vi "18.DMA-FIFO-2通道.vi"() -> ()   [LabVIEW 2019]
uses:
  <vilib>/rvi/Emulation/niFpgaGetClockAttributes.vi
  <vilib>/rvi/Emulation/niFpgaSctlEmulationGetInTimedLoop.vi
  <vilib>/rvi/Emulation/niFpgaEmulationReportErrorSimple.vi
  <vilib>/rvi/eio/common/nirviEmuTemplateMethod_errors.vi
  <vilib>/rvi/interface/RandomDataEmulation/niFpgaRandomDataHandleErrors.vi
  <vilib>/rvi/Emulation/niFpgaProcessEmulError.vi
  <vilib>/rvi/Emulation/niFpgaCriticalErrorInLSC.vi
  <vilib>/eio/EIONode/EIONode.xnode
  <vilib>/rvi/DataTransferAndStorage/Container/XNode/niFpgaContainer.xnode
  <vilib>/rvi/interface/RandomDataEmulation/nirviRandomDataFpgaReadWriteTemplate.vi
panel:
  in  "stop":bool
  in  "DMA Cleared?":bool
  out "Overflow?":bool
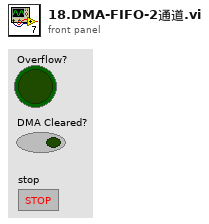
[diagram p1: front panel]
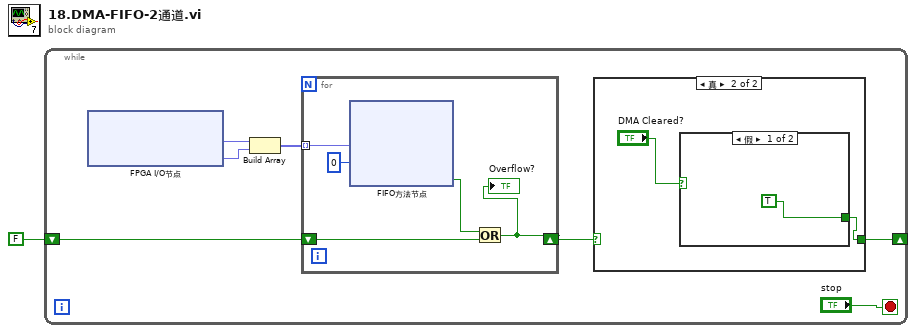
[diagram p0: block diagram]
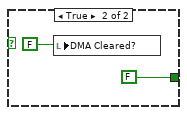
[diagram p3: hidden frame]
diagram:
  n1 = while {
    shift-right: [w3] -> _
    shift-left: FALSE -> [w5]
    stop <- "stop" stop-if-true
    n2 = xnode "FPGA I/O节点"() -> ("ConnectorB/AI0"=w8:fxp<+/-,24,5>, "ConnectorB/AI1"=w7:fxp<+/-,24,5>)  [unwired: 2 in, 2 out]
    n3 = Build Array(w8, w7) -> (w6:fxp<+/-,24,5>[])
    n4 = for {
      tunnel: w6 -> [w19] mode=indexing
      shift-right: [w15] -> w4
      shift-left: w5 -> [w17]
      n5 = xnode ("FIFO方法节点")("元素"=w19, "超时"=0) -> ("超时？"=w16:bool)  [unwired: 1 in, 1 out]
      n6 = Or(x=w16, y=w17) -> (x .or. y?=w15:bool)
      "Overflow?" <- w15
    }
    n7 = case shown="真" w4 {
      selector: w4 -> [w9 _]
      tunnel: [w9 w10] -> w3
      frame False {
      }
      frame True {
        n8 = case shown="假" "DMA Cleared?" {
          tunnel: [TRUE FALSE] -> w10
          frame False {
          }
          frame True {
            n9 = local write "DMA Cleared?"(FALSE) -> ()
          }
        }
      }
    }
  }
